vi "Set Configuration.vi"(8 "error in (no error)":errorcluster, 10 "configuration":T1={"name"="Transfer"}, 11 "Core Transfers Configuration in":refnum<class "Transfer Configuration.lvclass">) -> (0 "error out":errorcluster, 3 "Core Transfers Configuration out":refnum<class "Transfer Configuration.lvclass">)   [LabVIEW 2019, in "DSF Core.lvlib" / "Transfer Configuration.lvclass"]
uses:
  Transfer Configuration.lvclass
  Typedefs/Core Transfer Configuration.ctl
  Transfer Configuration.lvclass/Transfer Configuration.ctl
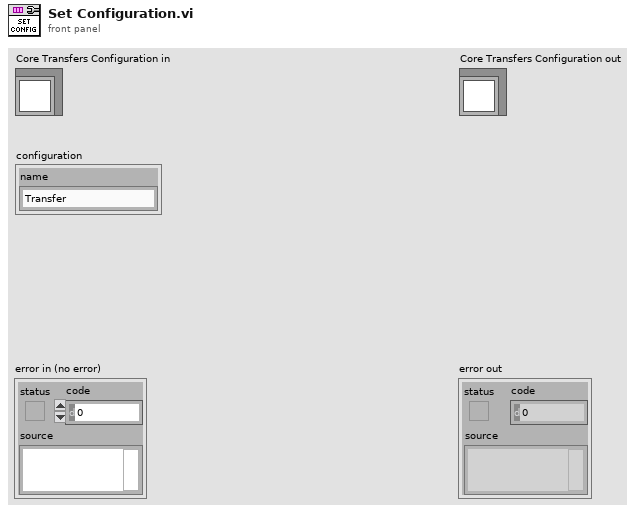
[diagram p1: front panel]
types:
  T1 = typedef "DSF Core.lvlib/Transfer Configuration.lvclass/Core Transfer Configuration.ctl" = cluster{"name":string}
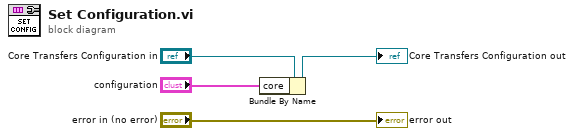
[diagram p0: block diagram]
diagram:
  n1 = Bundle By Name(cluster="Core Transfers Configuration in", "core"="configuration") -> (→"Core Transfers Configuration out":refnum<class "Transfer Configuration.lvclass">)
  "error out" <- "error in (no error)"
